vi "5790A_range.vi"(2 "error in":errorcluster, 3 "input voltage for range locking":dbl, 4 "range":enum32{"AUTO", "LOCK", "UP", "DOWN"}(ring), 5 "5790A":refnum<visa-resource-name>) -> (0 "error out":errorcluster, 1 "Session Out":refnum<visa-resource-name>)   [LabVIEW 2020]
uses:
  <vilib>/Instr/_visa.llb/VISA GPIB Control REN Mode.ctl
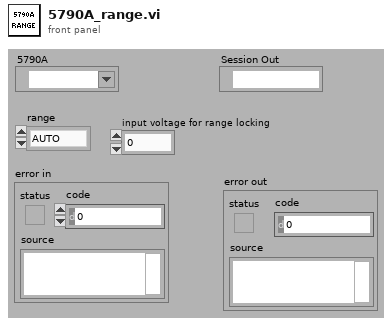
[diagram p1: front panel]
types:
  T1 = typedef "VISA GPIB Control REN Mode.ctl" = u16
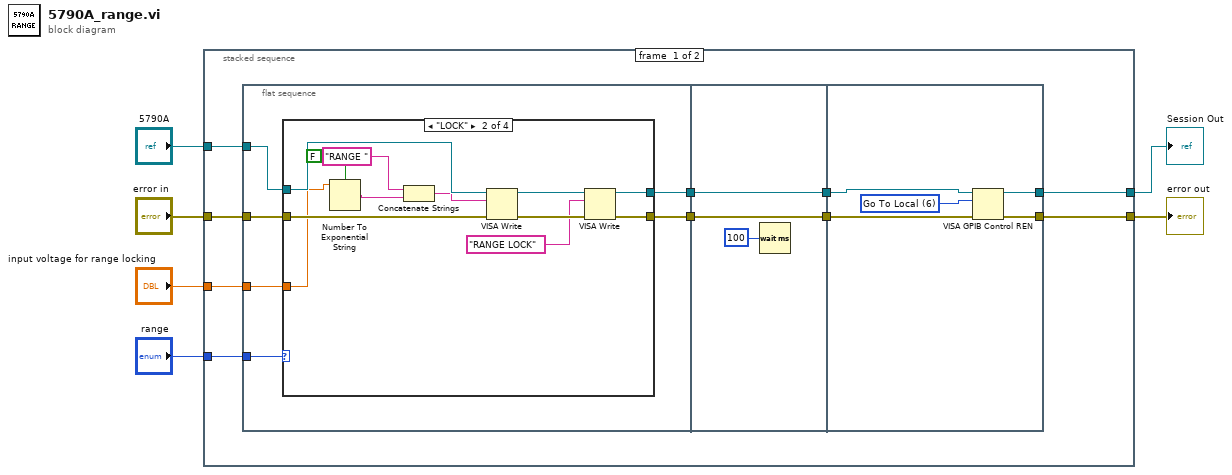
[diagram p0: block diagram]
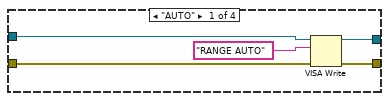
[diagram p2: hidden frame]
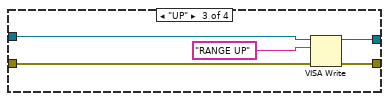
[diagram p3: hidden frame]
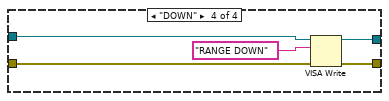
[diagram p4: hidden frame]
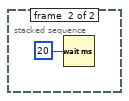
[diagram p5: hidden frame]
diagram:
  n1 = stacked-sequence {
    tunnel: "5790A" -> [w16 _]
    tunnel: "range" -> [w12 _]
    tunnel: [w15 _] -> w4
    tunnel: [w14 _] -> w5
    tunnel: "error in" -> [w13 _]
    tunnel: "input voltage for range locking" -> [w7 _]
    frame #0 {
      n2 = flat-sequence {
        tunnel: w16 -> [w20]
        tunnel: w13 -> [w21]
        tunnel: w12 -> [w22]
        tunnel: [w19] -> w11
        tunnel: [w18] -> w9
        tunnel: w7 -> [w17]
        tunnel: w11 -> [w52]
        tunnel: [w52] -> w10
        tunnel: w9 -> [w51]
        tunnel: [w51] -> w8
        tunnel: [w53] -> w14
        tunnel: [w54] -> w15
        tunnel: w10 -> [w55]
        tunnel: w8 -> [w56]
        frame #0 {
          n3 = case shown="\"LOCK\"" w22 {
            tunnel: w20 -> [w26 w39 w42 w48]
            tunnel: w21 -> [w24 w38 w41 w45]
            tunnel: [w25 w35 w44 w47] -> w18
            tunnel: [w23 w34 w40 w46] -> w19
            tunnel: w17 -> [_ w29 _ _]
            frame "AUTO" {
              n4 = VISA Write(VISA resource name=w26, write buffer="RANGE AUTO", error in (no error)=w24) -> (VISA resource name out=w25:refnum<visa-resource-name>, error out=w23:errorcluster)  [unwired: 1 out]
            }
            frame "LOCK" {
              n5 = Number To Exponential String(number=w29, 1:FALSE ("use system decimal point (T)")) -> (E-format string=w30:string)  [unwired: 2 in]
              n6 = Concatenate Strings("RANGE " ("string"), w30) -> (w32:string)
              n7 = VISA Write(VISA resource name=w39, write buffer=w32, error in (no error)=w38) -> (VISA resource name out=w37:refnum<visa-resource-name>, error out=w36:errorcluster)  [unwired: 1 out]
              n8 = VISA Write(VISA resource name=w37, write buffer="RANGE LOCK", error in (no error)=w36) -> (VISA resource name out=w35:refnum<visa-resource-name>, error out=w34:errorcluster)  [unwired: 1 out]
            }
            frame "UP" {
              n9 = VISA Write(VISA resource name=w42, write buffer="RANGE UP", error in (no error)=w41) -> (VISA resource name out=w44:refnum<visa-resource-name>, error out=w40:errorcluster)  [unwired: 1 out]
            }
            frame "DOWN" {
              n10 = VISA Write(VISA resource name=w48, write buffer="RANGE DOWN", error in (no error)=w45) -> (VISA resource name out=w47:refnum<visa-resource-name>, error out=w46:errorcluster)  [unwired: 1 out]
            }
          }
        }
        frame #1 {
          n11 = Wait (ms)(milliseconds to wait=u32 100) -> ()  [unwired: 1 out]
        }
        frame #2 {
          w57 = T1 6 items=["Deassert REN", "Assert REN", "Go To Local; Deassert REN ", "Assert REN; Address Device", "Local Lockout (Addressed Devices)", "Local Lockout (This Device)", "Go To Local"] ("Mode")
          n12 = VISA GPIB Control REN(8:w55, 10:w57, 11:w56) -> (0:w54:errorcluster, 3:w53:refnum<visa-resource-name>)
        }
      }
    }
    frame #1 {
      n13 = Wait (ms)(milliseconds to wait=u32 20 ("millisecond multiple")) -> ()  [unwired: 1 out]
    }
  }
  "Session Out" <- w5
  "error out" <- w4
